vi "Multirecord Acquisition Create.vi"(6 "DRAM":T1, 9 "instance":u8, 10 "acq.fetch fifo in":refnum<k21>, 11 "acq.status fifo in":refnum<k21>) -> (2 "acquisition resources":refnum<class "niInstr Multirecord Acquisition Common v1 FPGA.lvclass">, 3 "Address Space Collection out":refnum<class "Address Space Collection.lvclass">)   [LabVIEW 2021]
uses:
  <instrlib>/_niInstr/Multirecord Acquisition/Common/v1/FPGA/niInstr Multirecord Acquisition Common v1 FPGA.lvclass
  <instrlib>/_niInstr/Multirecord Acquisition/Common/v1/FPGA/Private/Create Resources DRAM U384x2 U768 Write Read.vi
  <instrlib>/_niInstr/Multirecord Acquisition/Common/v1/FPGA/Private/Create Fetch DMA FIFO Resources U8x32.vi
  <instrlib>/_niInstr/Instruction Framework/v1/FPGA/Interfaces/Address Space Collection/Address Space Collection.lvclass
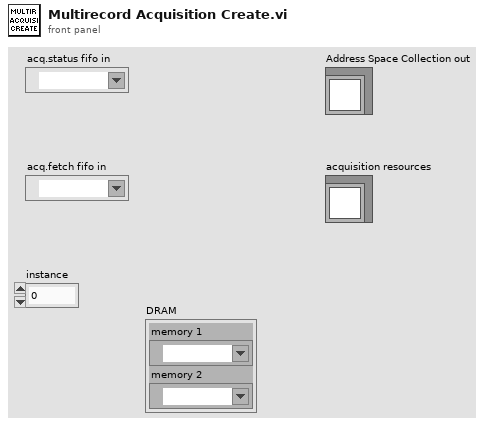
[diagram p1: front panel]
types:
  T1 = cluster{"memory 1":refnum<k21>, "memory 2":refnum<k21>}
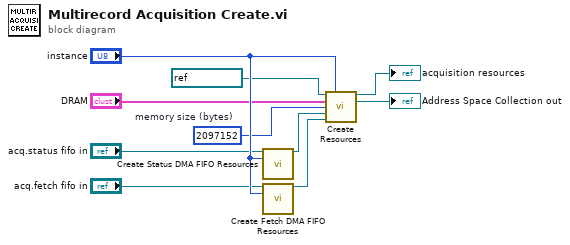
[diagram p0: block diagram]
diagram:
  w9 = u64 2097152  # memory size (bytes)
  n1 = call <instrlib>:"Create Status DMA FIFO Resources.vi"("status dma fifo in"="acq.status fifo in", "fifo instance"="instance") -> ("status dma fifo out"=w6:refnum<class "niInstr Status FIFO v1 FPGA.lvclass">)  [unwired: 13 in]
  n2 = call-poly <instrlib>:"Create Fetch DMA FIFO Resources.vi"("fetch dma fifo in"="acq.fetch fifo in", "fifo instance"="instance") -> ("fetch dma fifo out"=w2:refnum<class "niInstr Fetch FIFO v1 FPGA.lvclass">)  [unwired: 13 in]
  n3 = call-poly <instrlib>:"Create Resources.vi"("memory clock"=refnum<k21> "160MHz" ("process clock"), "instance"="instance", "memory"="DRAM", "memory size (bytes)"=w9, "status dma fifo resources"=w6, "fetch dma fifo resources"=w2) -> ("acquisition resources"=→"acquisition resources":refnum<class "niInstr Multirecord Acquisition Common v1 FPGA.lvclass">, "acquisition subsystem"=→"Address Space Collection out":refnum<class "Address Space Collection.lvclass">)  [unwired: 8 in]
